vi "SVPWMTestHarness.vi"() -> ()   [LabVIEW 2015]
uses:
  <vilib>/rvi/FXPMathLib/FxpSinAndCos/XNode/nifxpmath_SinAndCos.xnode
  <vilib>/rvi/FXPMathLib/FxpSinAndCos/simVIs/DllFxpSinAndCosTemp_sub.vi
  <vilib>/rvi/FXPMathLib/FxpSinAndCos/subVIs/nifxpmath_SinAndCos_SimConfig.ctl
  <vilib>/Platform/TimedLoop/XDataNode/XDataNode.xnode
  <vilib>/Platform/TimedLoop/XDataNode/nitl_modes.ctl
  <vilib>/Platform/TimedLoop/XDataNode/XDNodeRunTimeDep.lvlib
  <vilib>/Platform/TimedLoop/XDataNode/wakeup.ctl
  <vilib>/Platform/TimedLoop/XDataNode/timing_clust.ctl
  SVPWM/SVPWM_FXP.ctl
  SVPWM/SVPWM.lvlib
  SVPWM/SVPWM_SGL.ctl
  <vilib>/eio/EIONode/EIONode.xnode
  <vilib>/rvi/eio/common/nirviEmuTemplateMethod_errors.vi
  QuadratureEncoder/dev/QuadEnc/QuadEnc.lvlib
  SVPWM/SVPWMabcSGL.vi
  SVPWM/SVPWMabcFXP.vi
  SVPWM/SwitchPositions.ctl
  QuadratureEncoder/dev/QuadEnc/Parameters.ctl
  QuadratureEncoder/dev/QuadEnc/Output.ctl
panel:
  out "EncOutput":T1
  in  "EncParameters":T2
  in  "engauge":bool
  in  "Deadtime":u8
  in  "Period":u32=4000
  in  "enable":bool
  in  "Reset Enc":bool
  in  "FXP":bool
  out "Cs":sgl
  out "Bs":sgl
  out "As":sgl
  out "SectorSGL":u8
  out "SwitchPositionsSGL":T3
  out "C":fxp<+/-,32,4>
  out "B":fxp<+/-,32,4>
  out "A":fxp<+/-,32,4>
  out "SectorFXP":u8
  out "SwitchPositionsFXP":T3
  in  "Count(Ticks)":u32=400
  in  "modulation":fxp<+/-,16,2>=1.0
  in  "freq":sgl
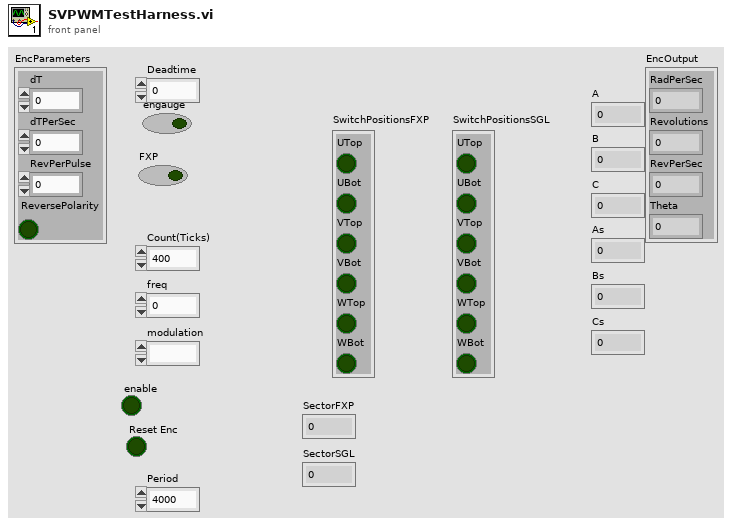
[diagram p1: front panel]
types:
  T1 = typedef "QuadEnc.lvlib/Output.ctl" = cluster{"RadPerSec":sgl, "Revolutions":sgl, "RevPerSec":sgl, "Theta":sgl}
  T2 = typedef "QuadEnc.lvlib/Parameters.ctl" = cluster{"dT":u32, "dTPerSec":sgl, "RevPerPulse":sgl, "ReversePolarity":bool}
  T3 = typedef "SVPWM.lvlib/SwitchPositions.ctl" = cluster{"UTop":bool, "UBot":bool, "VTop":bool, "VBot":bool, "WTop":bool, "WBot":bool}
  T4 = typedef "XDNodeRunTimeDep.lvlib/timing_clust.ctl" = cluster{"Expected End [f-1]":u64, "Actual End [f-1]":u64, "Finished Late? [f-1]":bool, "Expected End [i-1]":u64, "Actual End [i-1]":u64, "Finished Late? [i-1]":bool, "Expected Start [i]":u64, "Actual Start [i]":u64, "Expected Start [f]":u64, "Actual Start [f]":u64, "Source Name":string, "Structure Name":string, "Period":i64, "Deadline":i64, "Offset":i64, "Start":i64, "Priority":i32, "Timeout":i32, "Mode":T5, "Wakeup Reason":T6, "Error":errorcluster, "Source Type":string, "Secondary Source Type":string, "Global End Time":u64, "Global Start Time":u64, "Frame Duration":u64, "Iteration Duration":u64, "Assigned CPU":i32, "I/O Scan Engine Mode":u32}
  T5 = typedef "XDNodeRunTimeDep.lvlib/nitl_modes.ctl" = enum32{"No Change", "Process missed periods, maintain original phase", "Discard missed periods, maintain original phase", "Process missed periods, ignore original phase", "Discard missed periods, ignore original phase"}
  T6 = typedef "XDNodeRunTimeDep.lvlib/wakeup.ctl" = enum32{"Normal", "Aborted", "Asynchronous wakeup", "Timing source error", "Timed loop error", "Timeout"}
  T7 = typedef "SVPWM.lvlib/SVPWM_SGL.ctl" = cluster{"max":sgl, "Period":u32, "Deadtime":u8}
  T8 = typedef "SVPWM.lvlib/SVPWM_FXP.ctl" = cluster{"max":fxp<+/-,32,4>, "Period":u32, "Deadtime":u8}
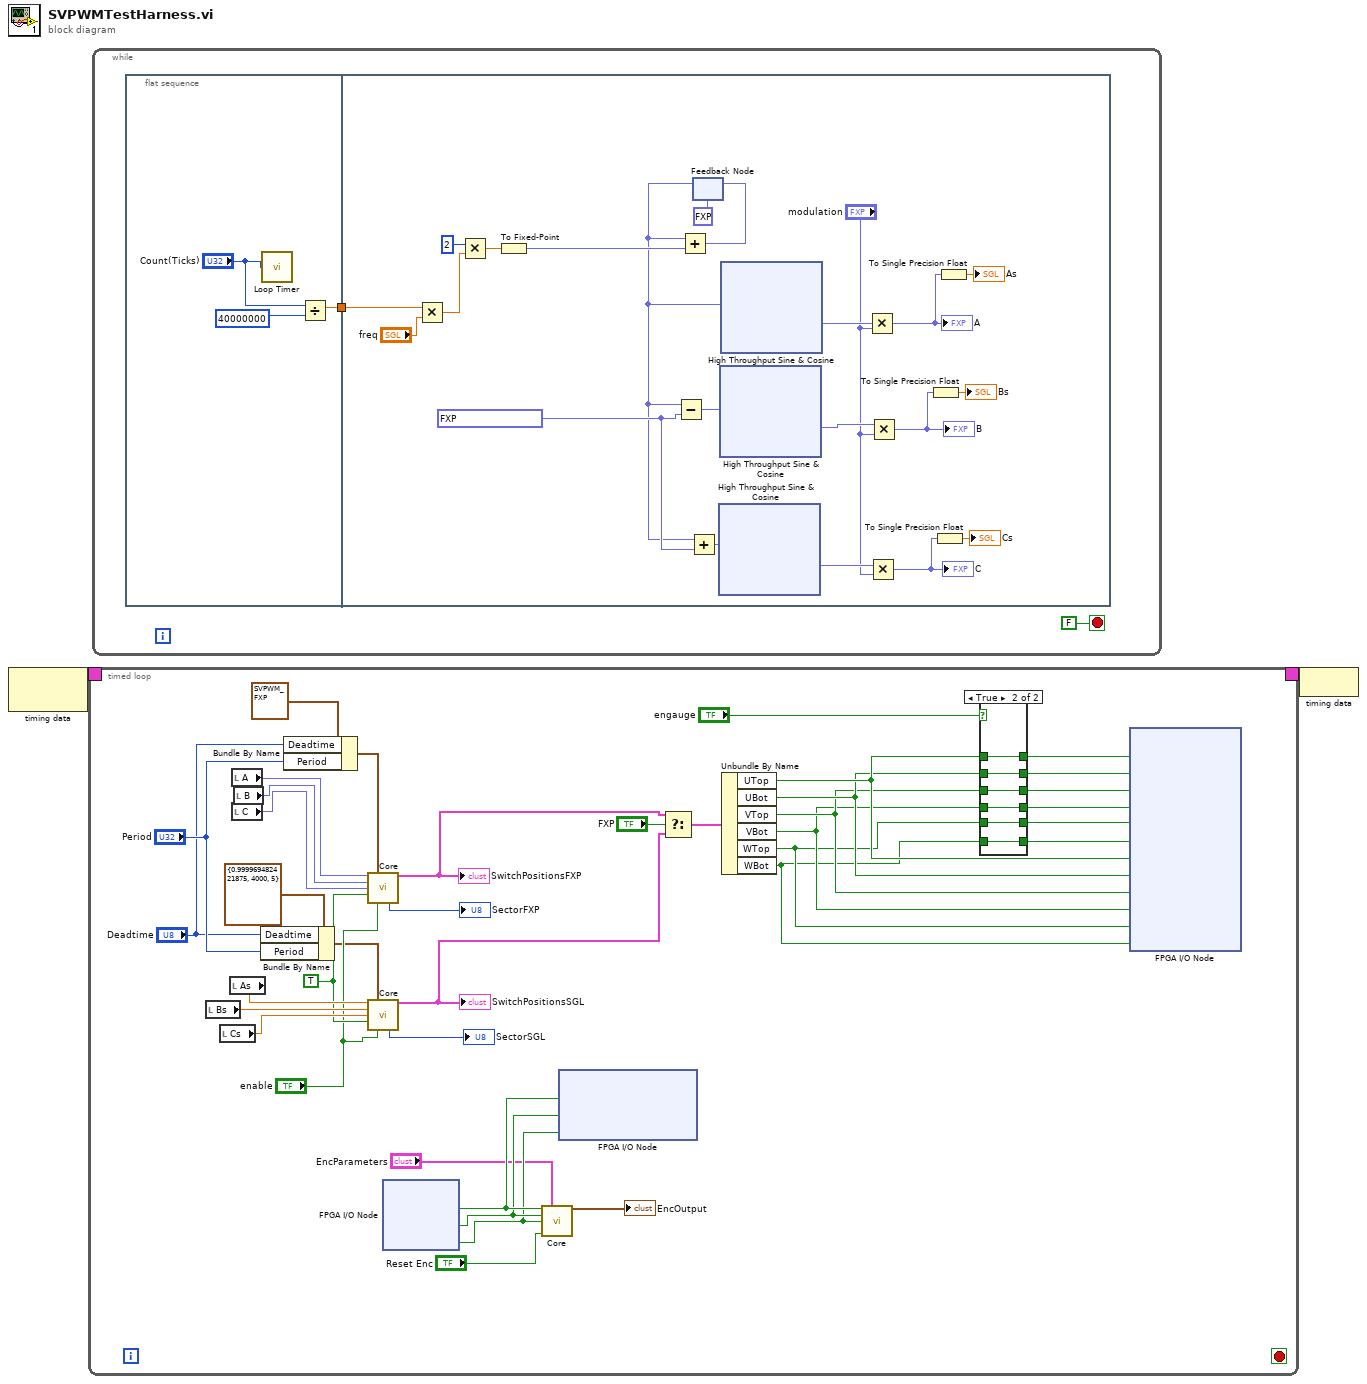
[diagram p0: block diagram]
diagram:
  n1 = node-c288() -> (w2:T4)  [unwired: 1 in]
  n2 = timed-loop {
    timing: w2 -> [_]
    timing-out: [_] -> w1
    stop <- _ stop-if-true
    w26 = TRUE ("enable")
    n3 = local read "Bs"() -> (w35:sgl)
    n4 = local read "Cs"() -> (w34:sgl)
    n5 = local read "As"() -> (w36:sgl)
    n6 = local read "A"() -> (w41:fxp<+/-,32,4>)
    n7 = local read "C"() -> (w39:fxp<+/-,32,4>)
    n8 = local read "B"() -> (w40:fxp<+/-,32,4>)
    n9 = Bundle By Name(cluster=T7 {"max"=0.9999695, "Period"=4000, "Deadtime"=5} ("SVPWM_SGL"), "Deadtime"="Deadtime", "Period"="Period") -> (w20:T7)
    n10 = Bundle By Name(cluster=T8 {"max"=0.999969482421875, "Period"=4000, "Deadtime"=5} ("SVPWMparams"), "Deadtime"="Deadtime", "Period"="Period") -> (w23:T8)
    n11 = call-poly "Core.vi"("A"=w41, "SVPWMparams"=w23, "B"=w40, "C"=w39, "input valid"=w26, "enable"="enable") -> ("SwitchPositions"=w32:T3, "Sector"=→"SectorFXP":u8)  [unwired: 7 in, 1 out]
    "SwitchPositionsFXP" <- w32
    n12 = call-poly "Core.vi"("A"=w36, "SVPWM_SGL"=w20, "B"=w35, "C"=w34, "input valid"=w26, "enable"="enable") -> ("SwitchPositions"=w31:T3, "Sector"=→"SectorSGL":u8)  [unwired: 7 in, 1 out]
    "SwitchPositionsSGL" <- w31
    n13 = xnode "FPGA I/O Node"() -> ("Enc_A"=w29:bool, "Enc_B"=w28:bool, "Enc_Z"=w27:bool)  [unwired: 3 in, 3 out]
    n14 = call "Core.vi"("A"=w29, "Parameters"="EncParameters", "B"=w28, "Z"=w27, "reset"="Reset Enc") -> ("Output"=→"EncOutput":T1)  [unwired: 7 in, 3 out]
    n15 = xnode "FPGA I/O Node"("GPIC/LVTTL/DIO3"=w29, "GPIC/LVTTL/DIO4"=w28, "GPIC/LVTTL/DIO5"=w27) -> ()  [unwired: 3 in, 3 out]
    n16 = Select(t=w32, s="FXP", f=w31) -> (s? t:f=w30:T3)
    n17 = Unbundle By Name(w30) -> ("UTop"=w17:bool, "UBot"=w15:bool, "VTop"=w13:bool, "VBot"=w11:bool, "WTop"=w9:bool, "WBot"=w7:bool)
    n18 = case shown="True" "engauge" {
      tunnel: w17 -> [_ w47]
      tunnel: [_ w47] -> w16
      tunnel: w15 -> [_ w46]
      tunnel: [_ w46] -> w14
      tunnel: w13 -> [_ w45]
      tunnel: [_ w45] -> w12
      tunnel: w11 -> [_ w44]
      tunnel: [_ w44] -> w10
      tunnel: w9 -> [_ w43]
      tunnel: [_ w43] -> w8
      tunnel: w7 -> [_ w42]
      tunnel: [_ w42] -> w6
      frame False {
      }
      frame True {
      }
    }
    n19 = xnode "FPGA I/O Node"("s2B / uTOPB"=w16, "s1B / uBOTB"=w14, "s4B / vTOPB"=w12, "s3B  / vBOTB"=w10, "s6B / wTOPB"=w8, "s5B / wBOTB"=w6, "uTOPB"=w17, "uBOTB"=w15, "vTOPB"=w13, "vBOTB"=w11, "wTOPB"=w9, "wBOTB"=w7) -> ()  [unwired: 12 in, 12 out]
  }
  n20 = while {
    stop <- FALSE stop-if-true
    n21 = flat-sequence {
      tunnel: [w52] -> w50
      tunnel: w50 -> [w68]
      frame #0 {
        n22 = call "Loop Timer"("Count(Ticks)"="Count(Ticks)") -> ()  [unwired: 1 out]
        n23 = Divide(x="Count(Ticks)", y=u32 40000000) -> (x/y=w52:sgl)
      }
      frame #1 {
        w75 = fxp<+/-,16,1> 0.666656494140625 ("x (pi)")
        n24 = Multiply(x=w68, y="freq") -> (x*y=w70:sgl)
        n25 = Multiply(x=i16 2, y=w70) -> (x*y=w57:sgl)
        n26 = To Fixed-Point(number=w57) -> (fixed-point=w56:fxp<+/-,32,16>)  [unwired: 1 in]
        n27 = feedback #1(fxp<+/-,16,1> 0.0 ("x (pi)")) -> (w55:fxp<+/-,16,1>)
        n28 = Subtract(x=w55, y=w75) -> (x-y=w74:fxp<+/-,17,2>)
        n29 = Add(x=w55, y=w56) -> (x+y=w71:fxp<+/-,16,1>)
        n30 = Add(x=w55, y=w75) -> (x+y=w76:fxp<+/-,17,2>)
        n31 = feedback-in #1(w71) -> ()
        n32 = xnode "High Throughput Sine & Cosine"("x (pi)"=w76) -> ("sin(x)"=w66:fxp<+/-,16,2>)  [unwired: 1 out]
        n33 = xnode "High Throughput Sine & Cosine"("x (pi)"=w74) -> ("sin(x)"=w65:fxp<+/-,16,2>)  [unwired: 1 out]
        n34 = xnode "High Throughput Sine & Cosine"("x (pi)"=w55) -> ("sin(x)"=w67:fxp<+/-,16,2>)  [unwired: 1 out]
        n35 = Multiply(x=w67, y="modulation") -> (x*y=w63:fxp<+/-,32,4>)
        "A" <- w63
        n36 = Multiply(x=w66, y="modulation") -> (x*y=w58:fxp<+/-,32,4>)
        "C" <- w58
        n37 = Multiply(x=w65, y="modulation") -> (x*y=w60:fxp<+/-,32,4>)
        "B" <- w60
        n38 = To Single Precision Float(number=w60) -> (single precision float=→"Bs":sgl)
        n39 = To Single Precision Float(number=w58) -> (single precision float=→"Cs":sgl)
        n40 = To Single Precision Float(number=w63) -> (single precision float=→"As":sgl)
      }
    }
  }
  n41 = node-c288(w1) -> ()
